vi "go_to_value.vi"(8 "error in":errorcluster, 10 "Target Value":dbl, 11 "address":string) -> (0 "error out":errorcluster)   [LabVIEW 2020]
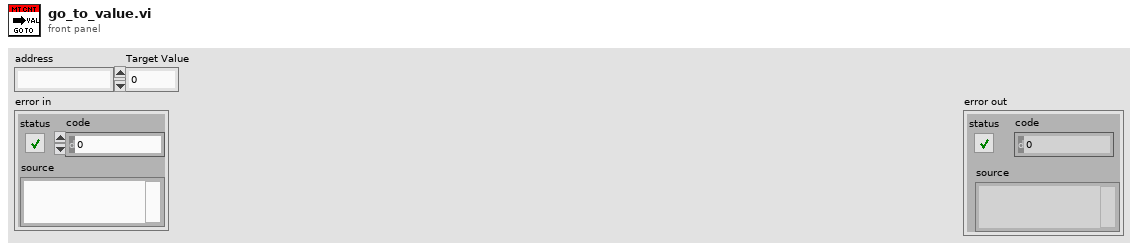
[diagram p1: front panel]
types:
  T1 = enum16{"Standard", "Buffered", "CRLF", "Immediate"}
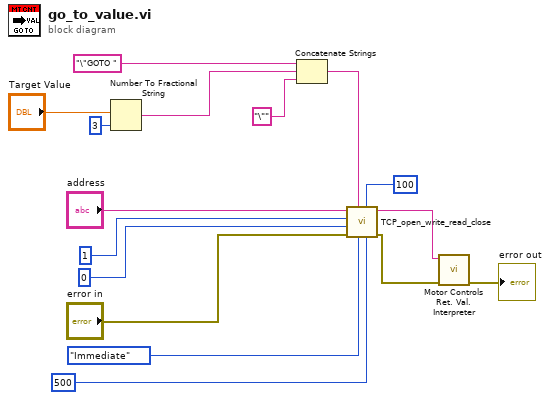
[diagram p0: block diagram]
diagram:
  n1 = Number To Fractional String(number="Target Value", precision (6)=i16 3) -> (F-format string=w3:string)  [unwired: 2 in]
  n2 = Concatenate Strings("\"GOTO " ("write string"), w3, "\"" ("string")) -> (w9:string)
  n3 = call "TCP_open_write_read_close.vi"("timeout ms (25000)"=500, "bytes to read"=100, "mode (standard)"=T1."Immediate", "write string"=w9, "error in"="error in", "local port (0)"=u16 0, "remote port or service name"=u16 1, "address"="address") -> ("error out"=w7:errorcluster, "read string"=w5:string)  [unwired: 2 in]
  n4 = call "Motor Controls Ret. Val. Interpreter.vi"("error in"=w7, "Command Return"=w5) -> ("error out"=→"error out":errorcluster)  [unwired: 8 in, 1 out]
